vi "Get String Value.vi"(6 "Default Value":string, 8 "error in (no error)":errorcluster, 10 "Name":string, 11 "Test Recipe in":refnum<class "Test Recipe.lvclass">) -> (0 "error out":errorcluster, 2 "Value":string, 3 "Test Recipe out":refnum<class "Test Recipe.lvclass">)   [LabVIEW 2015]
uses:
  Test Recipe.lvclass
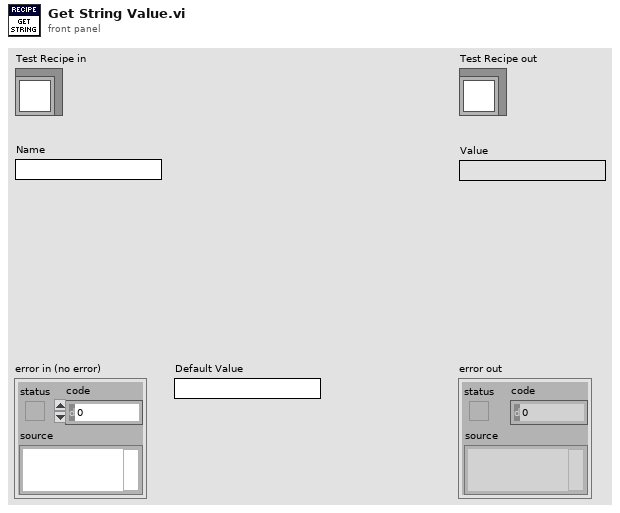
[diagram p1: front panel]
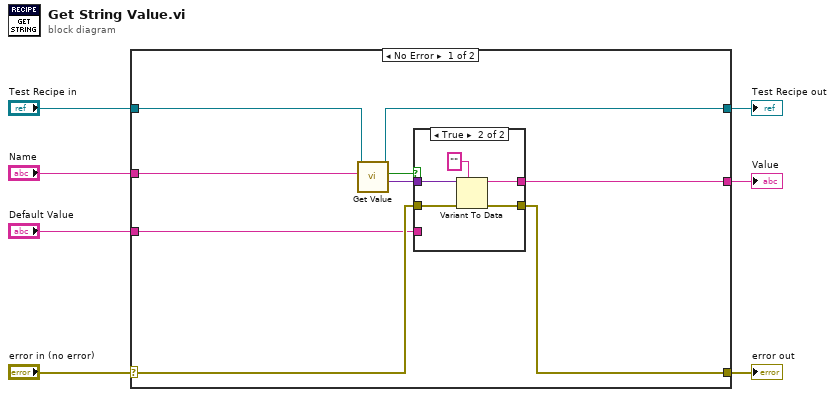
[diagram p0: block diagram]
diagram:
  n1 = case shown="No Error" "error in (no error)" {
    selector: "error in (no error)" -> [w11 w25]
    tunnel: [w10 w25] -> w6
    tunnel: [w15 w24] -> w4
    tunnel: "Test Recipe in" -> [w16 w24]
    tunnel: "Name" -> [w14 _]
    tunnel: [w12 _] -> w2
    tunnel: "Default Value" -> [w8 _]
    frame No Error {
      n2 = call-dynamic "Get Value.vi"("Key"=w14, "Registry in"=w16) -> ("Value"=w13:variant, "found?"=w9:bool, "Registry out"=w15:refnum<class "Test Recipe.lvclass">)  [unwired: 6 in, 1 out]
      n3 = case shown="True" w9 {
        tunnel: w13 -> [_ w23]
        tunnel: [w17 w22] -> w12
        tunnel: w11 -> [w18 w21]
        tunnel: [w18 w20] -> w10
        tunnel: w8 -> [w17 _]
        frame False {
        }
        frame True {
          n4 = Variant To Data(error in=w21, type="", Variant=w23) -> (data=w22:string, error out=w20:errorcluster)
        }
      }
    }
    frame Error {
    }
  }
  "error out" <- w6
  "Test Recipe out" <- w4
  "Value" <- w2
